vi "ModbusMotorDriver.vi"(9 "Mode":bool, 10 "M;otor Speed Controls":T4, 11 "Motor Bool Control":T5) -> (0 "error IO":errorcluster, 1 "Read Speed":T3 {"ReadSpeed2" format="%.2f"; "ReadSpeed1" format="%.2f"; "SetSpeed2" format="%.2f"; "SetSpeed1" format="%.2f"}, 2 "Motor Status Indicators":T1, 3 "Motor Bool Control Indicators":T2, 5 "register values":u16[](array[numeric]))   [LabVIEW 2024]
uses:
  support/MotorBoolControls.ctl
  support/MotorSpeedControls.ctl
  support/ReadSpeed.ctl
  support/MotorBoolControlsIndicators.ctl
  support/MotorStatusIndicators.ctl
panel:
  in  "stop":bool
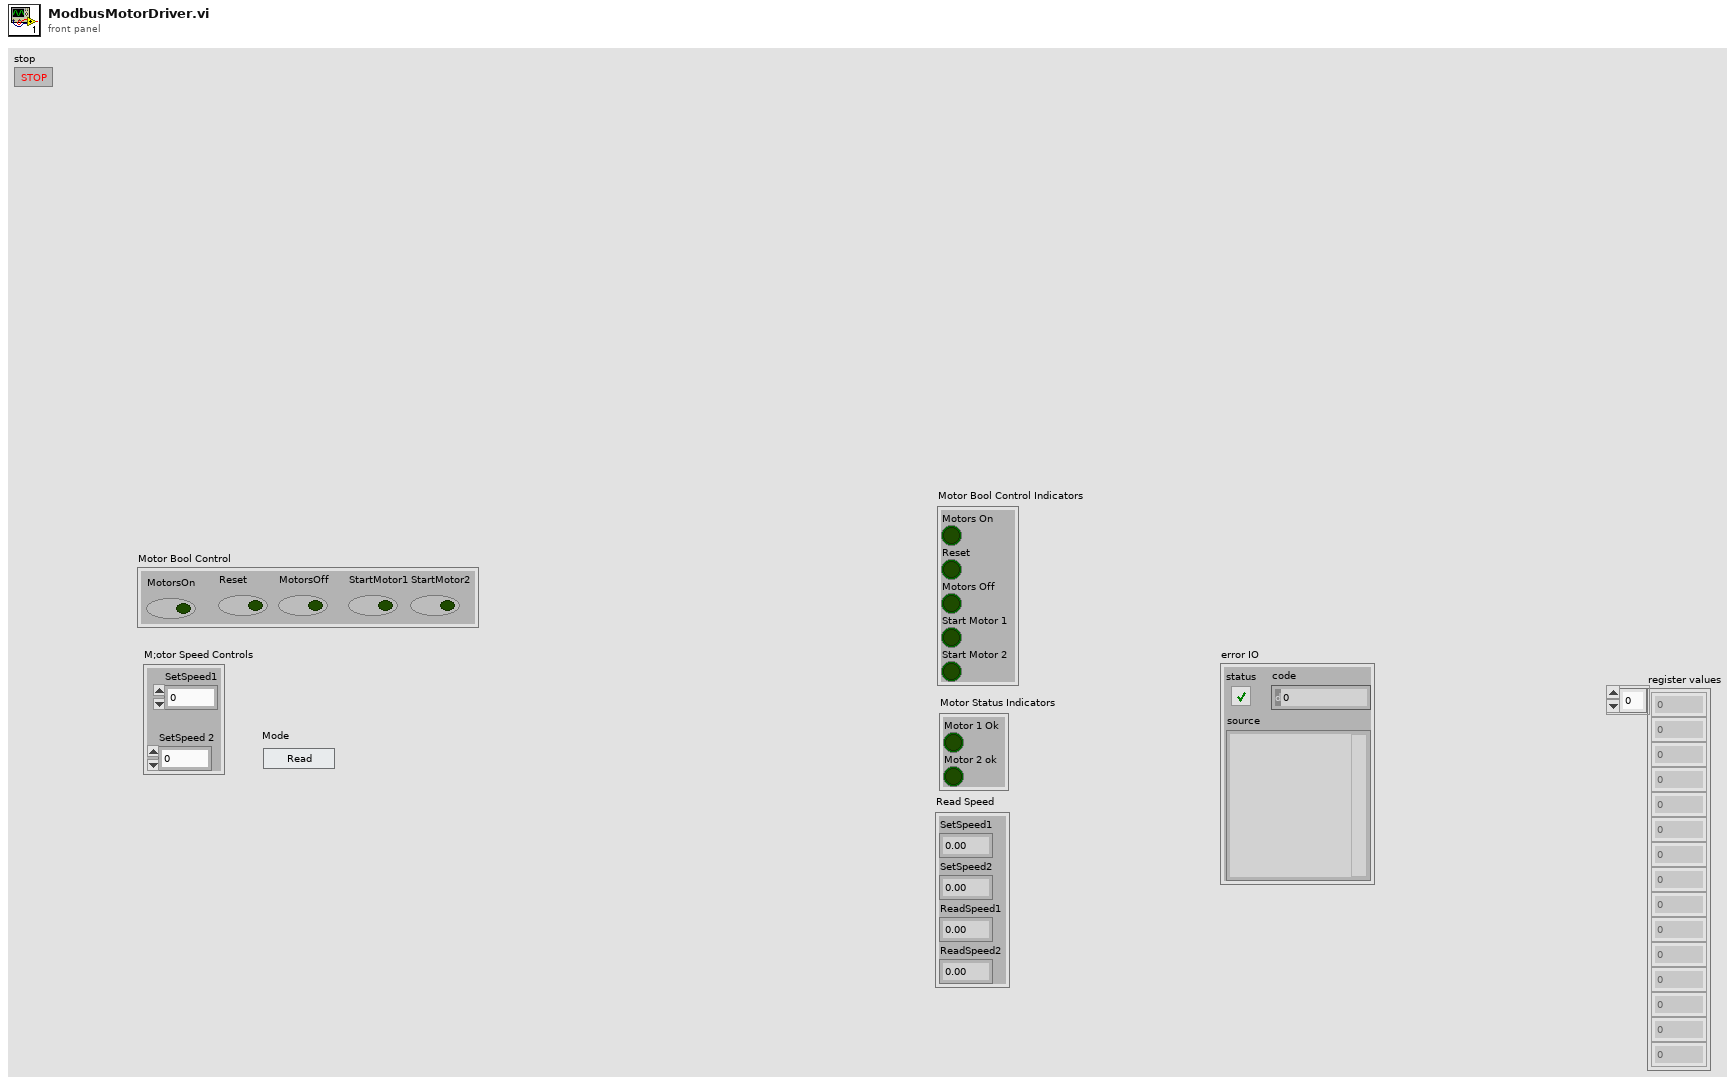
[diagram p1: front panel]
types:
  T1 = typedef "MotorStatusIndicators.ctl" = cluster{"Motor 1 Ok":bool, "Motor 2 ok":bool}
  T2 = typedef "MotorBoolControlsIndicators.ctl" = cluster{"Motors On":bool, "Reset":bool, "Motors Off":bool, "Start Motor 1 ":bool, "Start Motor 2":bool}
  T3 = typedef "ReadSpeed.ctl" = cluster{"SetSpeed1":dbl, "SetSpeed2":dbl, "ReadSpeed1":dbl, "ReadSpeed2":dbl}
  T4 = typedef "MotorSpeedControls.ctl" = cluster{"SetSpeed1":dbl, "SetSpeed 2":dbl}
  T5 = typedef "MotorBoolControls.ctl" = cluster{"MotorsOn":bool, "Reset":bool, "MotorsOff":bool, "StartMotor1":bool, "StartMotor2":bool}
  T6 = cluster{"[0] Motor1On":bool, "[1]Motor2On":bool, "[6] MotorsOff":bool, "[9]Motor1Ok":bool, "[10]Motor2Ok":bool}
  T7 = cluster{"[2]StartMotor1":bool, "[3]StartMotor2":bool}
  T8 = cluster{"[4] SetSpeed1":dbl, "[5] SetSpeed2":dbl, "[7]ReadSpeed1":dbl, "[8] ReadSpeed2":dbl}
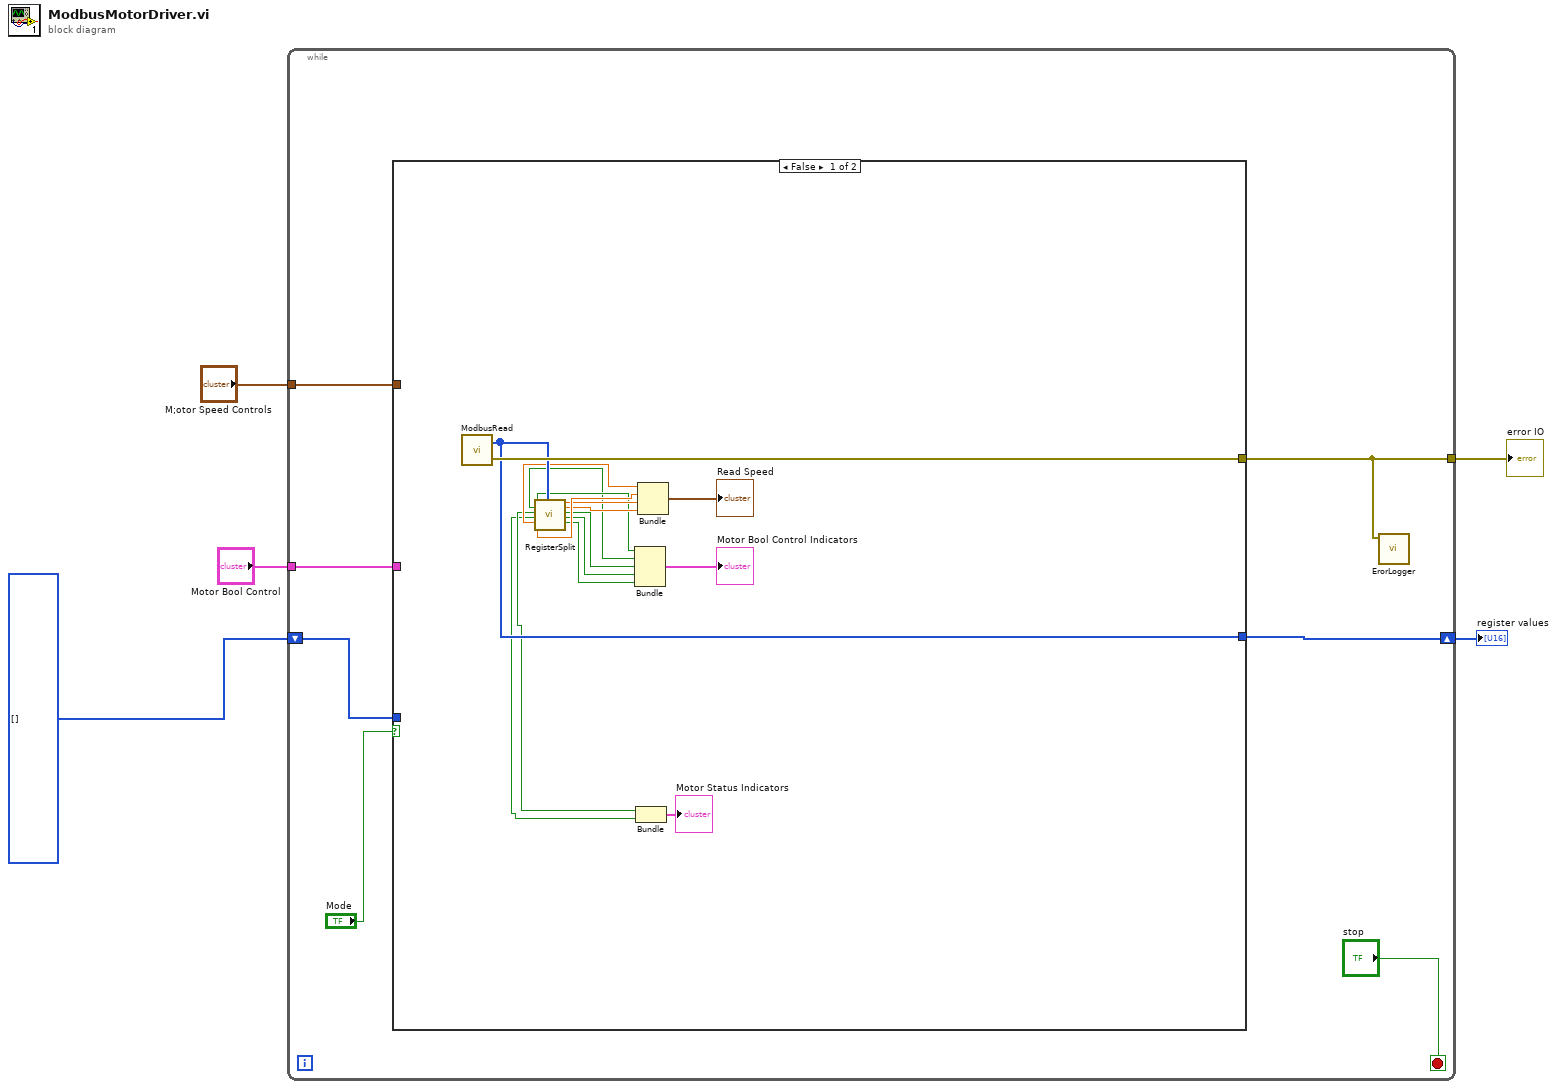
[diagram p0: block diagram]
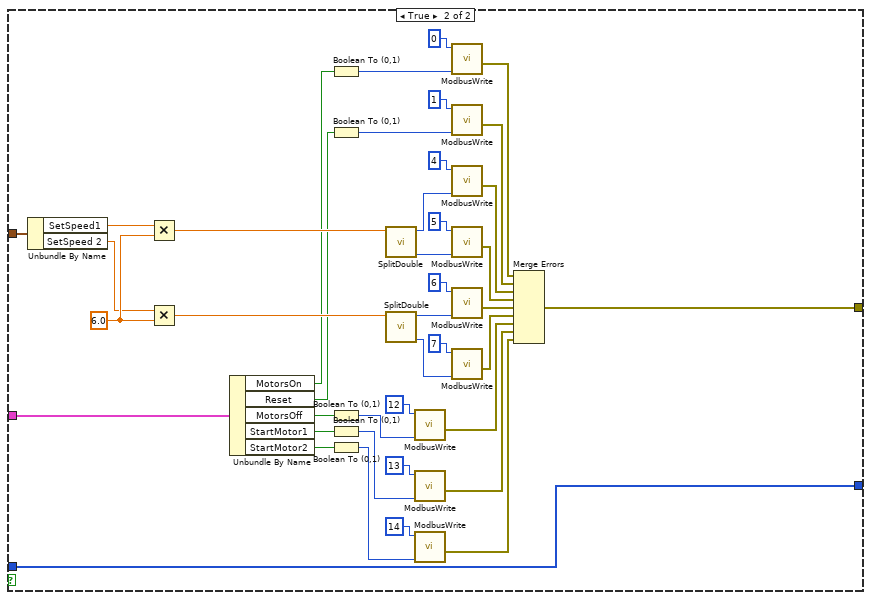
[diagram p2: hidden frame]
diagram:
  n1 = while {
    tunnel: "Motor Bool Control" -> [w11]
    tunnel: "M;otor Speed Controls" -> [w10]
    tunnel: [w8] -> w1
    shift-right: [w9] -> w2
    shift-left: u16[] [] ("register values") -> [w12]
    stop <- "stop" stop-if-true
    n2 = case shown="False" "Mode" {
      tunnel: [w28 w54] -> w8
      tunnel: [w27 w69] -> w9
      tunnel: w12 -> [_ w69]
      tunnel: w11 -> [_ w37]
      tunnel: w10 -> [_ w31]
      frame False {
        n3 = call "ModbusRead.vi"() -> ("error out"=w28:errorcluster, "register values"=w27:u16[])  [unwired: 2 in]
        n4 = call "RegisterSplit.vi"("register values"=w27) -> ("[0] Motor1On"=w21:bool, "[1]Motor2On"=w20:bool, "[2]StartMotor1"=w15:bool, "[3]StartMotor2"=w14:bool, "[4] SetSpeed1"=w26:dbl, "[5] SetSpeed2"=w25:dbl, "[7]ReadSpeed1"=w24:dbl, "[8] ReadSpeed2"=w23:dbl, "[6] MotorsOff"=w19:bool, "[9]Motor1Ok"=w18:bool, "[10]Motor2Ok"=w17:bool)  [unwired: 8 in]
        n5 = Bundle("[0] Motor1On"=w21, "[1]Motor2On"=w20, "[6] MotorsOff"=w19, "[9]Motor1Ok"=w18, "[10]Motor2Ok"=w17) -> (→"Motor Bool Control Indicators":T6)  [unwired: 1 in]
        n6 = Bundle("[2]StartMotor1"=w15, "[3]StartMotor2"=w14) -> (→"Motor Status Indicators":T7)  [unwired: 1 in]
        n7 = Bundle("[4] SetSpeed1"=w26, "[5] SetSpeed2"=w25, "[7]ReadSpeed1"=w24, "[8] ReadSpeed2"=w23) -> (→"Read Speed":T8)  [unwired: 1 in]
      }
      frame True {
        w38 = 6.0 ("y")
        n8 = Unbundle By Name(w31) -> ("SetSpeed1"=w30:dbl, "SetSpeed 2"=w29:dbl)
        n9 = Multiply(x=w30, y=w38) -> (x*y=w40:dbl)
        n10 = Multiply(x=w29, y=w38) -> (x*y=w39:dbl)
        n11 = Unbundle By Name(w37) -> ("MotorsOn"=w36:bool, "Reset"=w35:bool, "MotorsOff"=w34:bool, "StartMotor1"=w33:bool, "StartMotor2"=w32:bool)
        n12 = Boolean To (0,1)(Boolean=w36) -> (0, 1=w64:i16)
        n13 = Boolean To (0,1)(Boolean=w35) -> (0, 1=w65:i16)
        n14 = Boolean To (0,1)(Boolean=w34) -> (0, 1=w55:i16)
        n15 = Boolean To (0,1)(Boolean=w33) -> (0, 1=w45:i16)
        n16 = Boolean To (0,1)(Boolean=w32) -> (0, 1=w43:i16)
        n17 = call "SplitDouble.vi"("number"=w40) -> ("Low"=w61:i16, "High"=w63:i16)  [unwired: 9 in]
        n18 = call "SplitDouble.vi"("number"=w39) -> ("Low"=w58:i16, "High"=w60:i16)  [unwired: 9 in]
        n19 = call "ModbusWrite.vi"("address"=u16 12, "holding register value"=w55) -> ("error out"=w47:errorcluster)  [unwired: 7 in]
        n20 = call "ModbusWrite.vi"("address"=u16 13, "holding register value"=w45) -> ("error out"=w42:errorcluster)  [unwired: 7 in]
        n21 = call "ModbusWrite.vi"("address"=u16 14, "holding register value"=w43) -> ("error out"=w41:errorcluster)  [unwired: 7 in]
        n22 = call "ModbusWrite.vi"("address"=u16 0, "holding register value"=w64) -> ("error out"=w53:errorcluster)  [unwired: 7 in]
        n23 = call "ModbusWrite.vi"("address"=u16 1, "holding register value"=w65) -> ("error out"=w52:errorcluster)  [unwired: 7 in]
        n24 = call "ModbusWrite.vi"("address"=u16 4, "holding register value"=w63) -> ("error out"=w51:errorcluster)  [unwired: 7 in]
        n25 = call "ModbusWrite.vi"("address"=u16 5, "holding register value"=w61) -> ("error out"=w50:errorcluster)  [unwired: 7 in]
        n26 = call "ModbusWrite.vi"("address"=u16 6, "holding register value"=w60) -> ("error out"=w49:errorcluster)  [unwired: 7 in]
        n27 = call "ModbusWrite.vi"("address"=u16 7, "holding register value"=w58) -> ("error out"=w48:errorcluster)  [unwired: 7 in]
        n28 = Merge Errors(w53, w52, w51, w50, w49, w48, w47, w42, w41) -> (w54:errorcluster)
      }
    }
    n29 = call "ErorLogger.vi"("error in (no error)"=w8) -> ()  [unwired: 11 in]
  }
  "register values" <- w2
  "error IO" <- w1
